vi "CenterMouse.vi"(8 "error in (no error)":errorcluster, 11 "Input in":refnum<class "Input.lvclass">) -> (0 "error out":errorcluster, 3 "Input out":refnum<class "Input.lvclass">)   [LabVIEW 2015, in "Input.lvclass"]
uses:
  Input.lvclass
  User32.dll
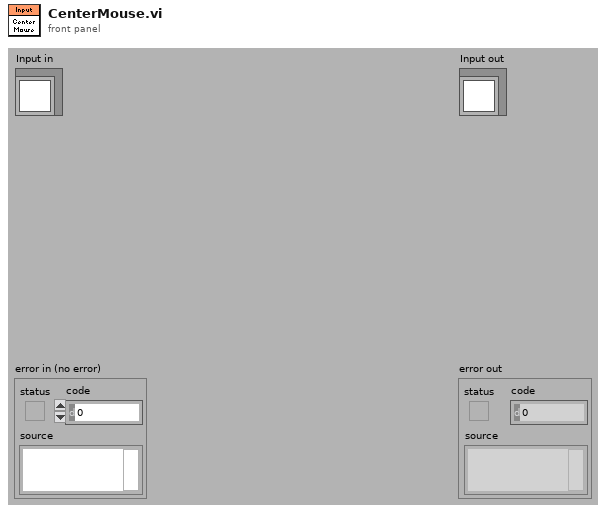
[diagram p1: front panel]
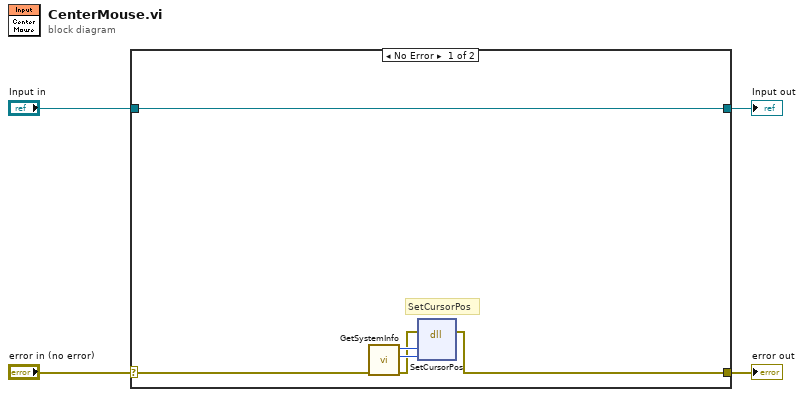
[diagram p0: block diagram]
diagram:
  n1 = case shown="No Error" "error in (no error)" {
    selector: "error in (no error)" -> [w6 w12]
    tunnel: [w9 w12] -> w3
    tunnel: [w10 w11] -> w1
    tunnel: "Input in" -> [w10 w11]
    frame No Error {
      # "SetCursorPos"
      n2 = call "GetSystemInfo.vi"("error in (no error)"=w6) -> ("error out"=w5:errorcluster, "Screen Y/2"=w7:i32, "Screen X/2"=w8:i32)  [unwired: 6 in, 2 out]
      n3 = dll-call lib="User32.dll" fn="SetCursorPos"(error in=w5, w8, w7) -> (error out=w9:errorcluster)  [unwired: 4 in, 2 out]
    }
    frame Error {
    }
  }
  "error out" <- w3
  "Input out" <- w1
